vi "Demo.vi"() -> ()   [LabVIEW 2018]
panel:
  in  "Demo?":bool
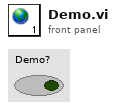
[diagram p1: front panel]
diagram:
